vi "Session Timeout--constant.vi"() -> (0 "Session Timeout (s)":dbl=300.0)   [LabVIEW 2016, in "WSsupport.lvlib"]
uses:
  WSsupport.lvlib
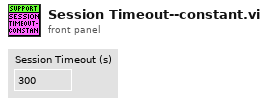
[diagram p1: front panel]
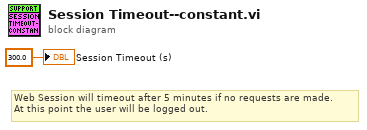
[diagram p0: block diagram]
diagram:
  # "Web Session will timeout after 5 minutes if no requests are made.\nAt this point the user will be logged out."
  "Session Timeout (s)" <- 300.0
